vi "PDash - New DQMH Unit Test.vi"(6 "Created Unit Test VI":path, 9 "Event Info":T1={"Event VI Path"=path "", "Argument Path"=path "", "Wait Argument Path"=path "", "Event Arg Owner"=-1, "Event Name"="", "Type"=enum."Request"}, 10 "Module Info":T3, 11 "Project":refnum<vi>) -> (0 "error out":errorcluster)   [LabVIEW 2019]
doc: "_____\nCreated using DQMH Event Scripter 7.1.0.1447."
uses:
  <vilib>/Delacor/Delacor QMH/Libraries/_Scripting Support/Module Info--cluster.ctl
  <vilib>/Delacor/Delacor QMH/Libraries/_Scripting Support/Module Type--enum.ctl
  <vilib>/Delacor/Delacor QMH/Libraries/_Scripting Support/Event Info (Unit Test)--cluster.ctl
  <vilib>/Delacor/Delacor QMH/Libraries/_Scripting Support/Event Type (Unit Test)--enum.ctl
  PantherDashboard Scripting Hooks/Panther Dasboard Scripting Hooks.lvlib
  <vilib>/Delacor/Delacor QMH/Libraries/_Scripting Support/dqmh_lib_DQMH Scripting Support.lvlib
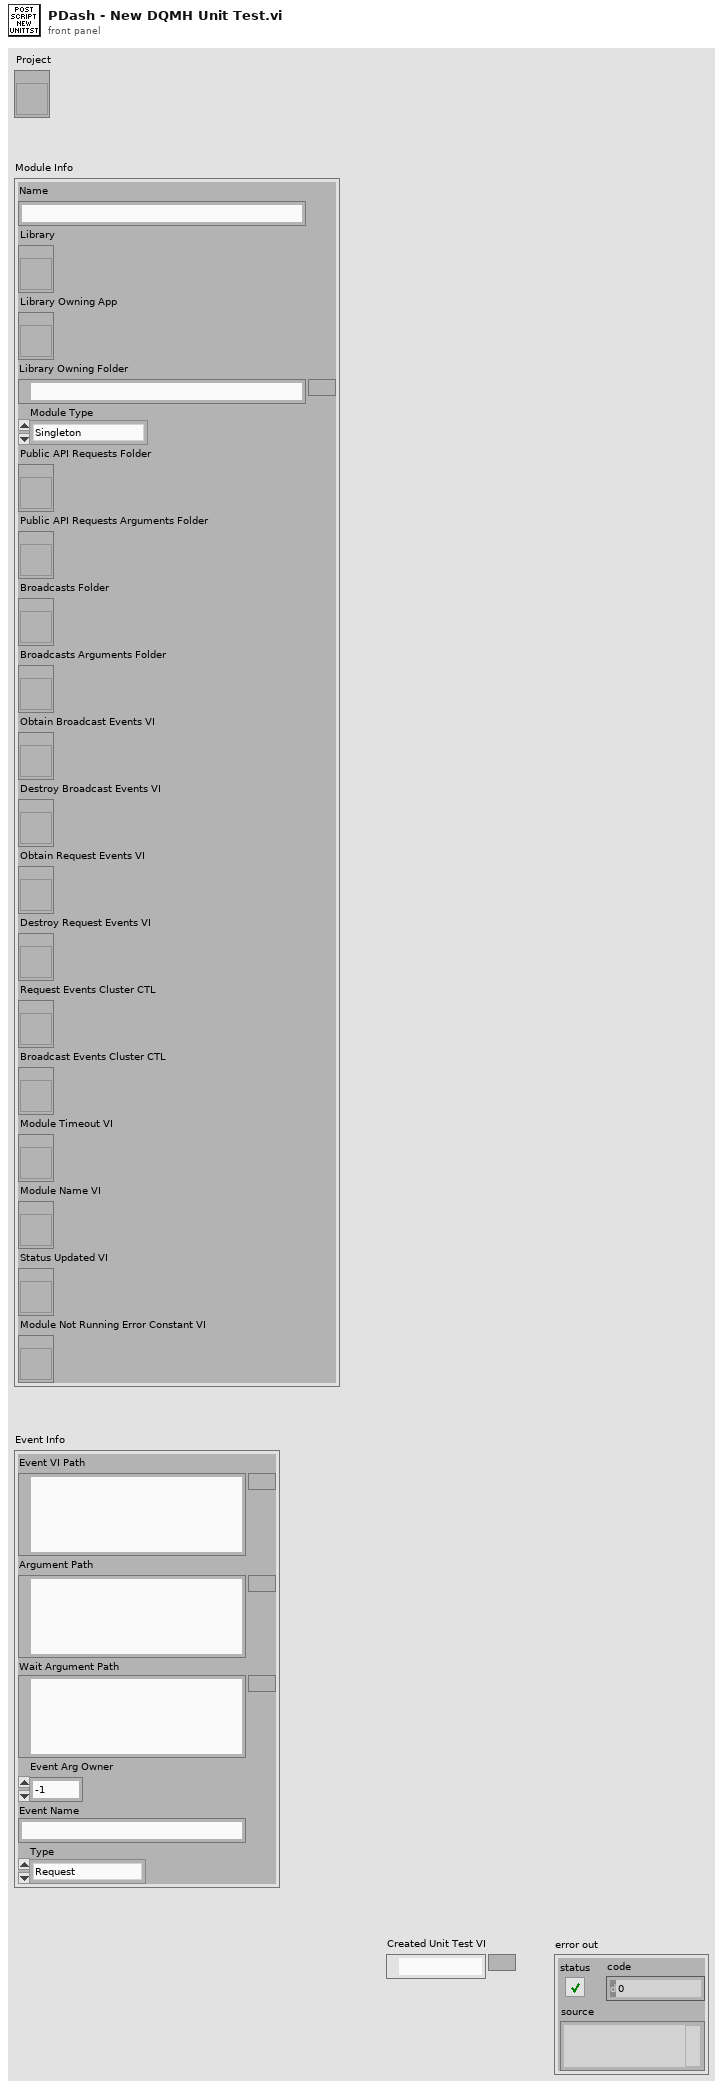
[diagram p1: front panel]
types:
  T1 = typedef "dqmh_lib_DQMH Scripting Support.lvlib/Event Info (Unit Test)--cluster.ctl" = cluster{"Event VI Path":path, "Argument Path":path, "Wait Argument Path":path, "Event Arg Owner":i32, "Event Name":string, "Type":T2}
  T2 = typedef "dqmh_lib_DQMH Scripting Support.lvlib/Event Type (Unit Test)--enum.ctl" = enum16{"Request", "Broadcast", "Both"}
  T3 = typedef "dqmh_lib_DQMH Scripting Support.lvlib/Module Info--cluster.ctl" = cluster{"Name":string, "Library":refnum<vi>, "Library Owning App":refnum<vi>, "Library Owning Folder":path, "Module Type":T4, "Public API Requests Folder":refnum<vi>, "Public API Requests Arguments Folder":refnum<vi>, "Broadcasts Folder":refnum<vi>, "Broadcasts Arguments Folder":refnum<vi>, "Obtain Broadcast Events VI":refnum<vi>, "Destroy Broadcast Events VI":refnum<vi>, "Obtain Request Events VI":refnum<vi>, "Destroy Request Events VI":refnum<vi>, "Request Events Cluster CTL":refnum<vi>, "Broadcast Events Cluster CTL":refnum<vi>, "Module Timeout VI":refnum<vi>, "Module Name VI":refnum<vi>, "Status Updated VI":refnum<vi>, "Module Not Running Error Constant VI":refnum<vi>}
  T4 = typedef "dqmh_lib_DQMH Scripting Support.lvlib/Module Type--enum.ctl" = enum16{"Singleton", "Cloneable"}
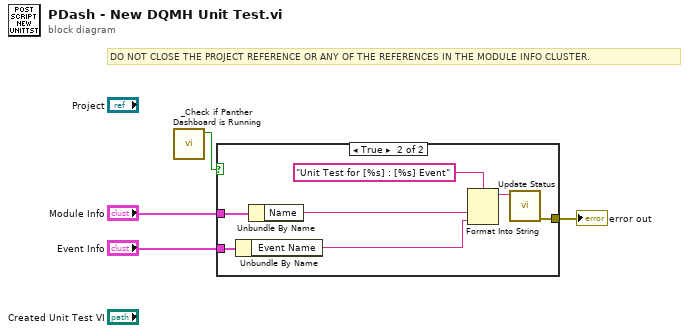
[diagram p0: block diagram]
diagram:
  # "DO NOT CLOSE THE PROJECT REFERENCE OR ANY OF THE REFERENCES IN THE MODULE INFO CLUSTER."
  n1 = call "_Check if Panther Dashboard is Running.vi"() -> ("Panther Dashboard is Running?"=w1:bool)  [unwired: 10 in, 1 out]
  n2 = case shown="True" w1 {
    tunnel: "Event Info" -> [_ w10]
    tunnel: [_ w11] -> w4
    tunnel: "Module Info" -> [_ w8]
    frame False {
    }
    frame True {
      n3 = Unbundle By Name(w10) -> ("Event Name"=w6:string)
      n4 = Unbundle By Name(w8) -> ("Name"=w7:string)
      n5 = Format Into String(format string="Unit Test for [%s] : [%s] Event", w7, w6) -> (resulting string=w5:string)  [unwired: 2 in, 1 out]
      n6 = call "_Update Status.vi"("Status"=w5) -> ("error out"=w11:errorcluster)  [unwired: 10 in]
    }
  }
  "error out" <- w4
